vi "Check Poistion Hall Pulse.vi"(8 "Segment Data":T2) -> (0 "Array":string[](array[string]), 2 "Segment Data 2":T2)   [LabVIEW 2018]
uses:
  type defs/Sequence Info.ctl
  type defs/Hall Pulse Range Control.ctl
panel:
  out "error out":errorcluster
  in  "Cluster":T1
  out "Name":string="Pre Run Station - Glass - Vent Open"
  in  "Description":string
  in  "Save":bool
  in  "Cancel":bool
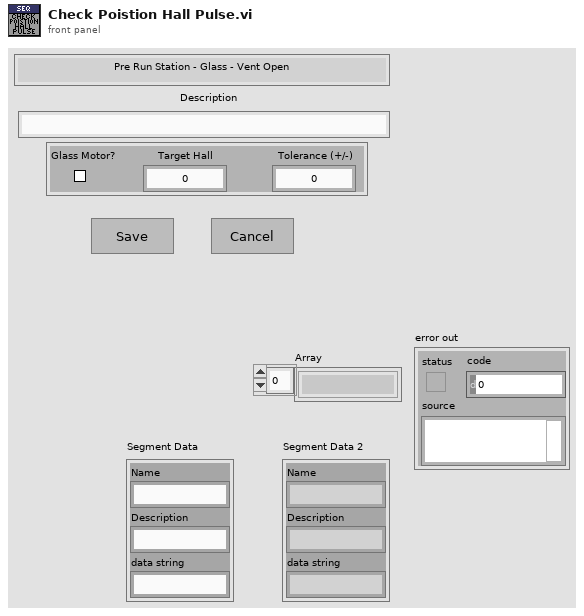
[diagram p1: front panel]
types:
  T1 = typedef "Hall Pulse Range Control.ctl" = cluster{"Target Hall":i32, "Tolerance (+/-)":u16, "Glass Motor?":bool}
  T2 = typedef "Sequence Info.ctl" = cluster{"Name":string, "Description":string, "data string":string}
  T3 = cluster{"Hall Pulse Range Control":T1, "Segment Data":T2, "Old Data":string, "New Data":string}
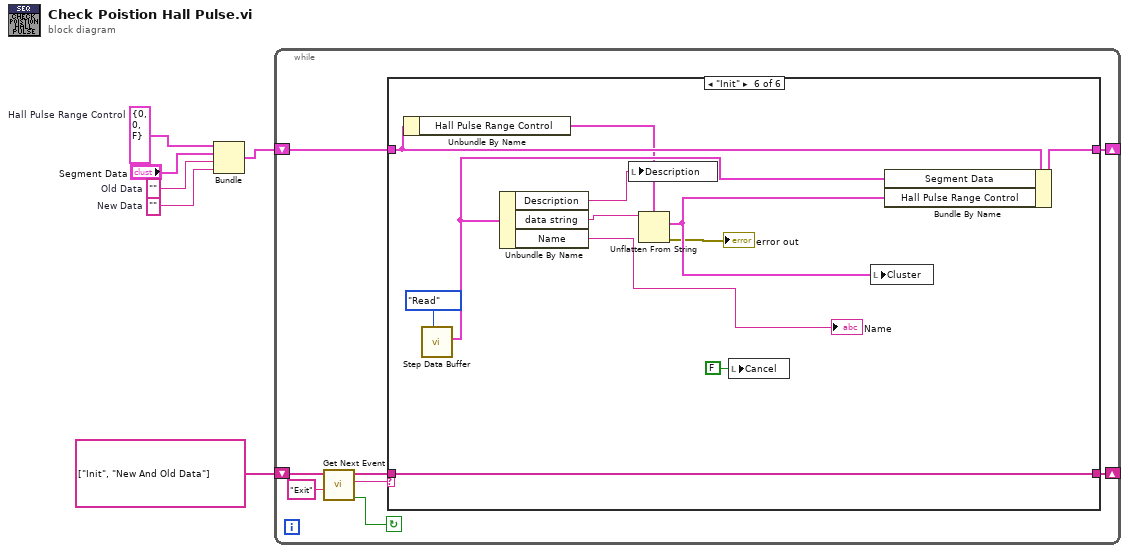
[diagram p0: block diagram]
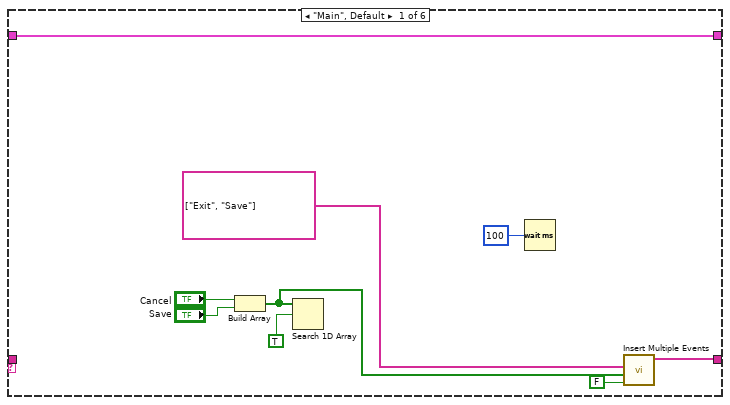
[diagram p2: hidden frame]
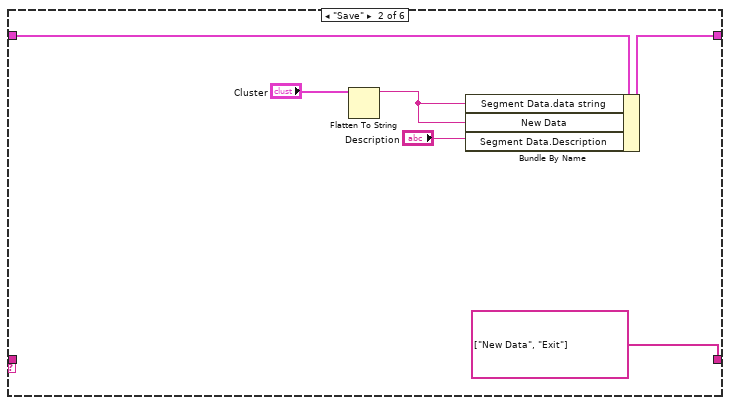
[diagram p3: hidden frame]
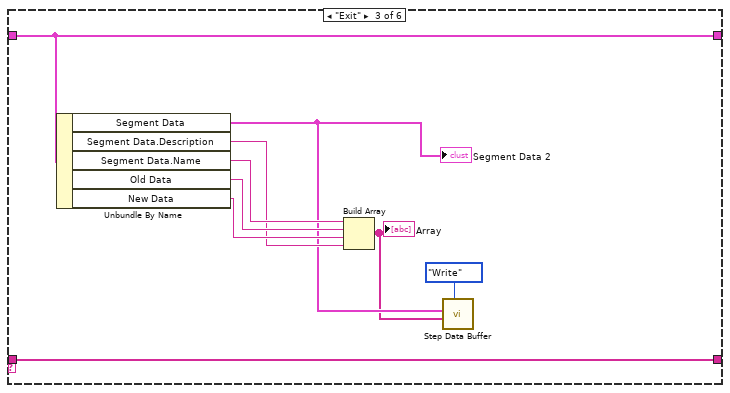
[diagram p4: hidden frame]
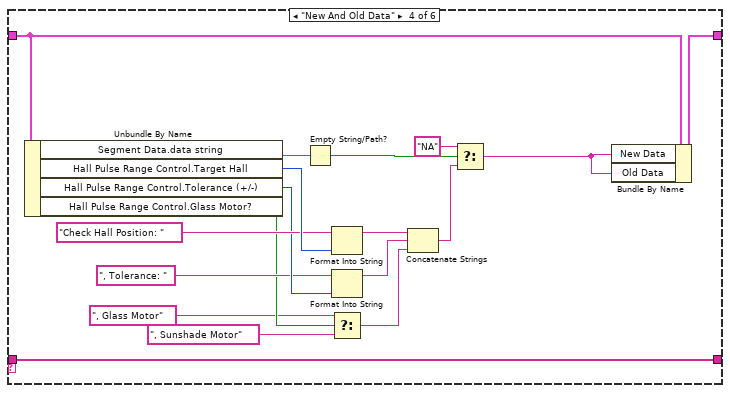
[diagram p5: hidden frame]
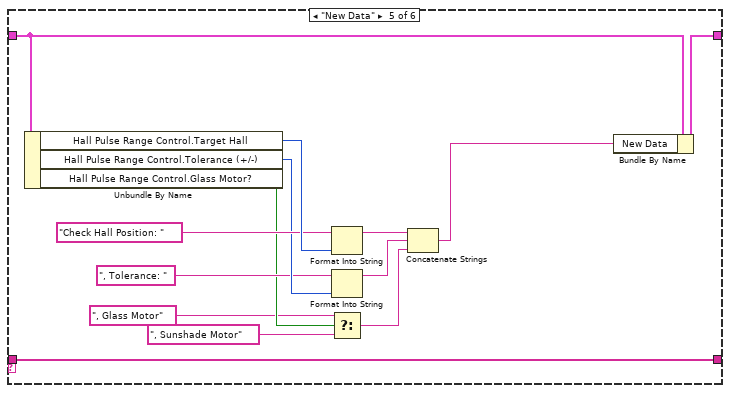
[diagram p6: hidden frame]
diagram:
  w1 = ""  # New Data
  w2 = ""  # Old Data
  w4 = T1 {"Target Hall"=0, "Tolerance (+/-)"=0, "Glass Motor?"=FALSE}  # Hall Pulse Range Control
  n1 = Bundle("Hall Pulse Range Control"=w4, "Segment Data"="Segment Data", "Old Data"=w2, "New Data"=w1) -> (w6:T3)  [unwired: 1 in]
  n2 = while {
    shift-right: [w12] -> _
    shift-left: string[] ["Init", "New And Old Data"] ("Event queue out") -> [w11]
    shift-right: [w7] -> _
    shift-left: w6 -> [w8]
    stop <- w10 continue-if-true
    n3 = call "Get Next Event.vi"("Exit Event"="Exit", "event queue in"=w11) -> ("Condition (Exit:F)"=w10:bool, "next event"=w14:string, "event queue out"=w13:string[])  [unwired: 3 in]
    n4 = case shown="\"Init\"" w14 {
      tunnel: w13 -> [_ _ w37 w56 w70 w81]
      tunnel: [w20 string[] ["New Data", "Exit"] ("Event queue out") w37 w56 w70 w81] -> w12
      tunnel: w8 -> [w15 w28 w38 w48 w66 w74]
      tunnel: [w15 w27 w38 w47 w65 w79] -> w7
      frame "Main", Default {
        n5 = Build Array("Cancel", "Save") -> (w18:bool[])
        n6 = Search 1D Array(1D array=w18, element=TRUE) -> ()  [unwired: 1 in, 1 out]
        n7 = Wait (ms)(milliseconds to wait=u32 100) -> ()  [unwired: 1 out]
        n8 = call "Insert Multiple Events.vi"("Insert all? (T)"=FALSE, "Insert Selected?"=w18, "Events to Insert"=string[] ["Exit", "Save"]) -> ("Event queue out"=w20:string[])  [unwired: 4 in]
      }
      frame "Save" {
        n9 = Flatten To String(anything="Cluster") -> (data string=w24:string)  [unwired: 3 in, 2 out]
        n10 = Bundle By Name(cluster=w28, "Segment Data.data string"=w24, "New Data"=w24, "Segment Data.Description"="Description") -> (w27:T3)
      }
      frame "Exit" {
        n11 = Unbundle By Name(w38) -> ("Segment Data"=w31:T2, "Segment Data.Description"=w33:string, "Segment Data.Name"=w36:string, "Old Data"=w35:string, "New Data"=w34:string)
        "Segment Data 2" <- w31
        n12 = Build Array(w36, w35, w34, w33) -> (w30:string[])
        "Array" <- w30
        n13 = call "Step Data Buffer.vi"("Mode"=enum16{"Init", "Read", "Write"}."Write", "Step Hisitory In"=w30, "Segment Data In"=w31) -> ()  [unwired: 4 in, 5 out]
      }
      frame "New And Old Data" {
        n14 = Unbundle By Name(w48) -> ("Segment Data.data string"=w55:string, "Hall Pulse Range Control.Target Hall"=w51:i32, "Hall Pulse Range Control.Tolerance (+/-)"=w46:u16, "Hall Pulse Range Control.Glass Motor?"=w44:bool)
        n15 = Empty String/Path?(string/path=w55) -> (empty?=w54:bool)
        n16 = Format Into String(initial string="Check Hall Position: ", w51) -> (resulting string=w49:string)  [unwired: 2 in, 1 out]
        n17 = Format Into String(initial string=", Tolerance: ", w46) -> (resulting string=w40:string)  [unwired: 2 in, 1 out]
        n18 = Select(t=", Glass Motor" ("initial string"), s=w44, f=", Sunshade Motor" ("initial string")) -> (s? t:f=w39:string)
        n19 = Concatenate Strings(w49, w40, w39) -> (w41:string)
        n20 = Select(t="NA", s=w54, f=w41) -> (s? t:f=w52:string)
        n21 = Bundle By Name(cluster=w48, "New Data"=w52, "Old Data"=w52) -> (w47:T3)
      }
      frame "New Data" {
        n22 = Unbundle By Name(w66) -> ("Hall Pulse Range Control.Target Hall"=w69:i32, "Hall Pulse Range Control.Tolerance (+/-)"=w64:u16, "Hall Pulse Range Control.Glass Motor?"=w62:bool)
        n23 = Format Into String(initial string="Check Hall Position: ", w69) -> (resulting string=w67:string)  [unwired: 2 in, 1 out]
        n24 = Format Into String(initial string=", Tolerance: ", w64) -> (resulting string=w59:string)  [unwired: 2 in, 1 out]
        n25 = Select(t=", Glass Motor" ("initial string"), s=w62, f=", Sunshade Motor" ("initial string")) -> (s? t:f=w58:string)
        n26 = Concatenate Strings(w67, w59, w58) -> (w57:string)
        n27 = Bundle By Name(cluster=w66, "New Data"=w57) -> (w65:T3)
      }
      frame "Init" {
        n28 = Unbundle By Name(w74) -> ("Hall Pulse Range Control"=w73:T1)
        n29 = call "Step Data Buffer.vi"("Mode"=enum16{"Init", "Read", "Write"}."Read") -> ("Segment Data Out"=w75:T2)  [unwired: 6 in, 4 out]
        n30 = Unbundle By Name(w75) -> ("Description"=w80:string, "data string"=w82:string, "Name"=→"Name":string)
        n31 = local write "Description"(w80) -> ()
        n32 = Unflatten From String(type=w73, binary string=w82) -> (value=w78:T1, error out=→"error out":errorcluster)  [unwired: 3 in, 1 out]
        n33 = local write "Cancel"(FALSE ("Cancel")) -> ()
        n34 = local write "Cluster"(w78) -> ()
        n35 = Bundle By Name(cluster=w74, "Segment Data"=w75, "Hall Pulse Range Control"=w78) -> (w79:T3)
      }
    }
  }
